vi "VMI_set_wave_list.vi"(5 "Table":string[][](table), 6 "Pump":dbl, 7 "Probe":dbl) -> (0 "Number delays":i32, 1 "Delay_list":dbl[][](array[numeric]), 2 "Delay_full_dir":string[](array[string]), 3 "First Point":dbl, 4 "Delay_dir_list":string[](array[string]))   [LabVIEW 2019]
panel:
  out "size(s)":i32[](array[numeric])
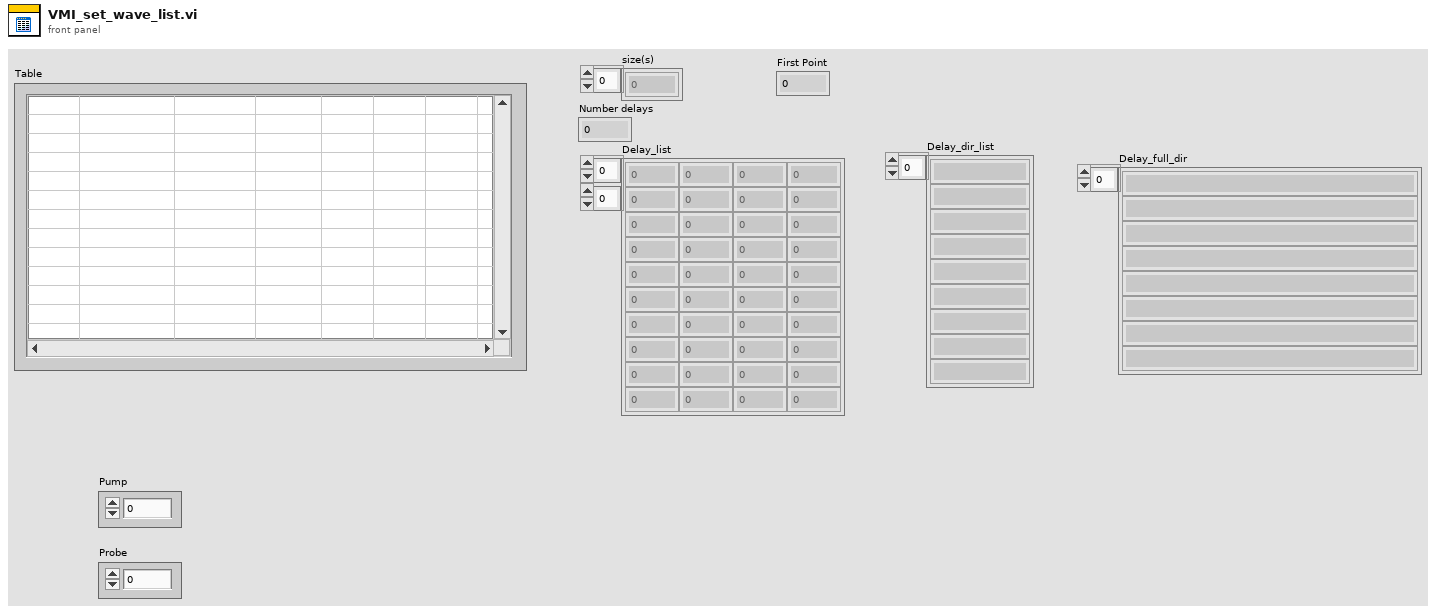
[diagram p1: front panel]
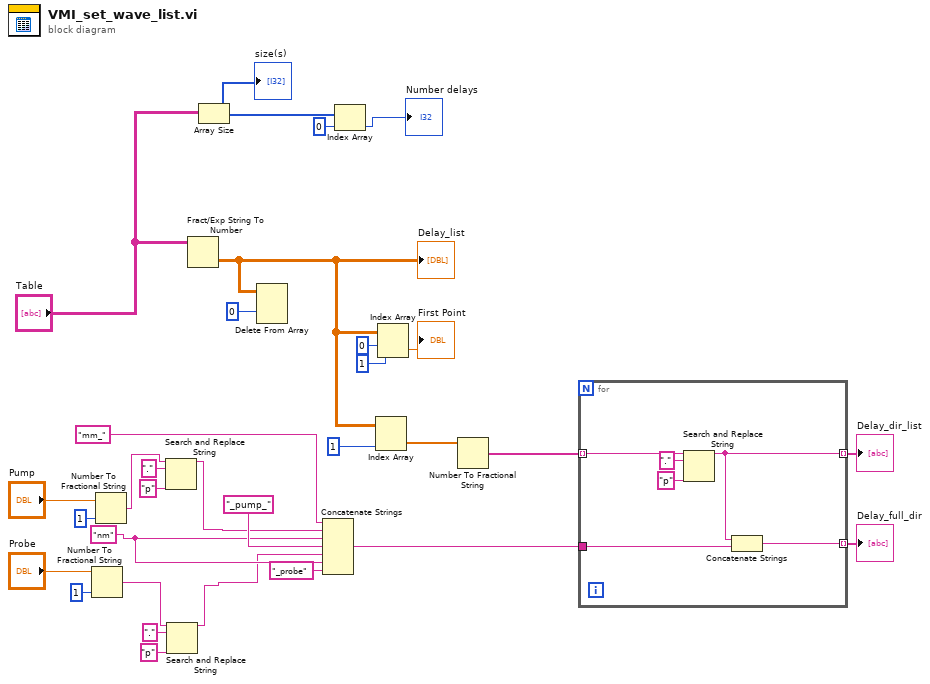
[diagram p0: block diagram]
diagram:
  w14 = "nm" ("string")
  n1 = Number To Fractional String(number="Probe", precision (6)=i16 1) -> (F-format string=w4:string)  [unwired: 2 in]
  n2 = Number To Fractional String(number="Pump", precision (6)=i16 1) -> (F-format string=w8:string)  [unwired: 2 in]
  n3 = Search and Replace String(input string=w8, search string=".", replace string="p" ("replace string (\"\")")) -> (result string=w7:string)  [unwired: 5 in, 3 out]
  n4 = Search and Replace String(input string=w4, search string=".", replace string="p" ("replace string (\"\")")) -> (result string=w3:string)  [unwired: 5 in, 3 out]
  n5 = Fract/Exp String To Number(string="Table") -> (number=w2:dbl[][])  [unwired: 3 in, 1 out]
  "Delay_list" <- w2
  n6 = Array Size(array="Table") -> (size(s)=w31:i32[])
  "size(s)" <- w31
  n7 = Delete From Array(array=w2, index (row)=0) -> ()  [unwired: 2 in, 2 out]
  n8 = Concatenate Strings("mm_", w7, w14, "_pump_" ("string"), w3, w14, "_probe" ("string")) -> (w12:string)
  n9 = Index Array(array=w31, index=0) -> (element=→"Number delays":i32)
  n10 = Index Array(array=w2, index (col)=1 ("index (row)")) -> (element=w23:dbl[])  [unwired: 1 in]
  n11 = Index Array(array=w2, index (row)=0, index (col)=1 ("disabled index (col)")) -> (element=→"First Point":dbl)
  n12 = Number To Fractional String(number=w23) -> (F-format string=w22:string[])  [unwired: 3 in]
  n13 = for {
    tunnel: w22 -> [w37] mode=indexing
    tunnel: [w33] -> w21 mode=indexing
    tunnel: w12 -> [w34]
    tunnel: [w32] -> w11 mode=indexing
    n14 = Search and Replace String(input string=w37, search string=".", replace string="p" ("replace string (\"\")")) -> (result string=w33:string)  [unwired: 5 in, 3 out]
    n15 = Concatenate Strings(w33, w34) -> (w32:string)
  }
  "Delay_dir_list" <- w21
  "Delay_full_dir" <- w11
